vi "Read key value pairs.vi"(8 "error in":errorcluster, 11 "fixed channel configuration in":refnum<class "fixed channel configuration.lvclass">) -> (0 "error out":errorcluster, 2 "key value pairs":string[][](array[string]), 3 "fixed channel configuration out":refnum<class "fixed channel configuration.lvclass">)   [LabVIEW 2013, in "fixed channel configuration.lvclass"]
uses:
  fixed channel configuration.lvclass
  fixed channel configuration.lvclass/fixed channel configuration.ctl
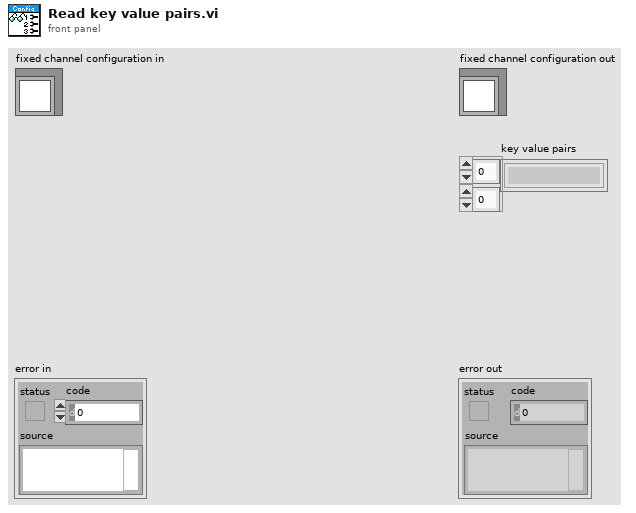
[diagram p1: front panel]
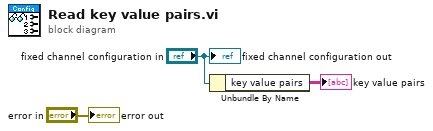
[diagram p0: block diagram]
diagram:
  n1 = Unbundle By Name("fixed channel configuration in") -> ("key value pairs"=→"key value pairs":string[][])
  "error out" <- "error in"
  "fixed channel configuration out" <- "fixed channel configuration in"
